vi "Aux2 IO.vi"() -> ()   [LabVIEW 2020]
uses:
  <vilib>/Platform/TimedLoop/XDataNode/timing_clust.ctl
  <vilib>/Platform/TimedLoop/XDataNode/nitl_modes.ctl
  <vilib>/Platform/TimedLoop/XDataNode/wakeup.ctl
  <vilib>/rvi/Emulation/niFpgaGetClockAttributes.vi
  <vilib>/rvi/Emulation/niFpgaSctlEmulationGetInTimedLoop.vi
  <vilib>/rvi/Emulation/niFpgaEmulationReportErrorSimple.vi
  <vilib>/rvi/eio/common/nirviEmuTemplateMethod_errors.vi
  <vilib>/rvi/Emulation/niFpgaProcessEmulError.vi
  <vilib>/rvi/Emulation/niFpgaCriticalErrorInLSC.vi
  <vilib>/eio/EIONode/EIONode.xnode
  <vilib>/platform/TimedLoop/XDataNode/XDataNode.xnode
  <vilib>/Platform/TimedLoop/XDataNode/XDNodeRunTimeDep.lvlib
  Front Panel Globals.vi
panel:
  out "Universal Data":sgl[](array[numeric])
  out "Universal Looprate":sgl
  out "TC Data":sgl[](array[numeric])
  out "TC Looprate":sgl
  out "RTD Data":sgl[](array[numeric])
  out "RTD Looprate":sgl
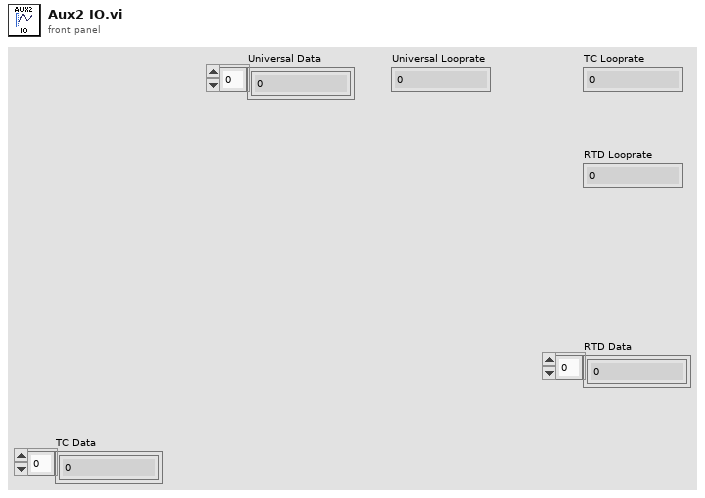
[diagram p1: front panel]
types:
  T1 = typedef "XDNodeRunTimeDep.lvlib/timing_clust.ctl" = cluster{"Expected End [f-1]":u64, "Actual End [f-1]":u64, "Finished Late? [f-1]":bool, "Expected End [i-1]":u64, "Actual End [i-1]":u64, "Finished Late? [i-1]":bool, "Expected Start [i]":u64, "Actual Start [i]":u64, "Expected Start [f]":u64, "Actual Start [f]":u64, "Source Name":string, "Structure Name":string, "Period":i64, "Deadline":i64, "Offset":i64, "Start":i64, "Priority":i32, "Timeout":i32, "Mode":T2, "Wakeup Reason":T3, "Error":errorcluster, "Source Type":string, "Secondary Source Type":string, "Global End Time":u64, "Global Start Time":u64, "Frame Duration":u64, "Iteration Duration":u64, "Assigned CPU":i32, "I/O Scan Engine Mode":u32}
  T2 = typedef "XDNodeRunTimeDep.lvlib/nitl_modes.ctl" = enum32{"No Change", "Process missed periods, maintain original phase", "Discard missed periods, maintain original phase", "Process missed periods, ignore original phase", "Discard missed periods, ignore original phase"}
  T3 = typedef "XDNodeRunTimeDep.lvlib/wakeup.ctl" = enum32{"Normal", "Aborted", "Asynchronous wakeup", "Timing source error", "Timed loop error", "Timeout"}
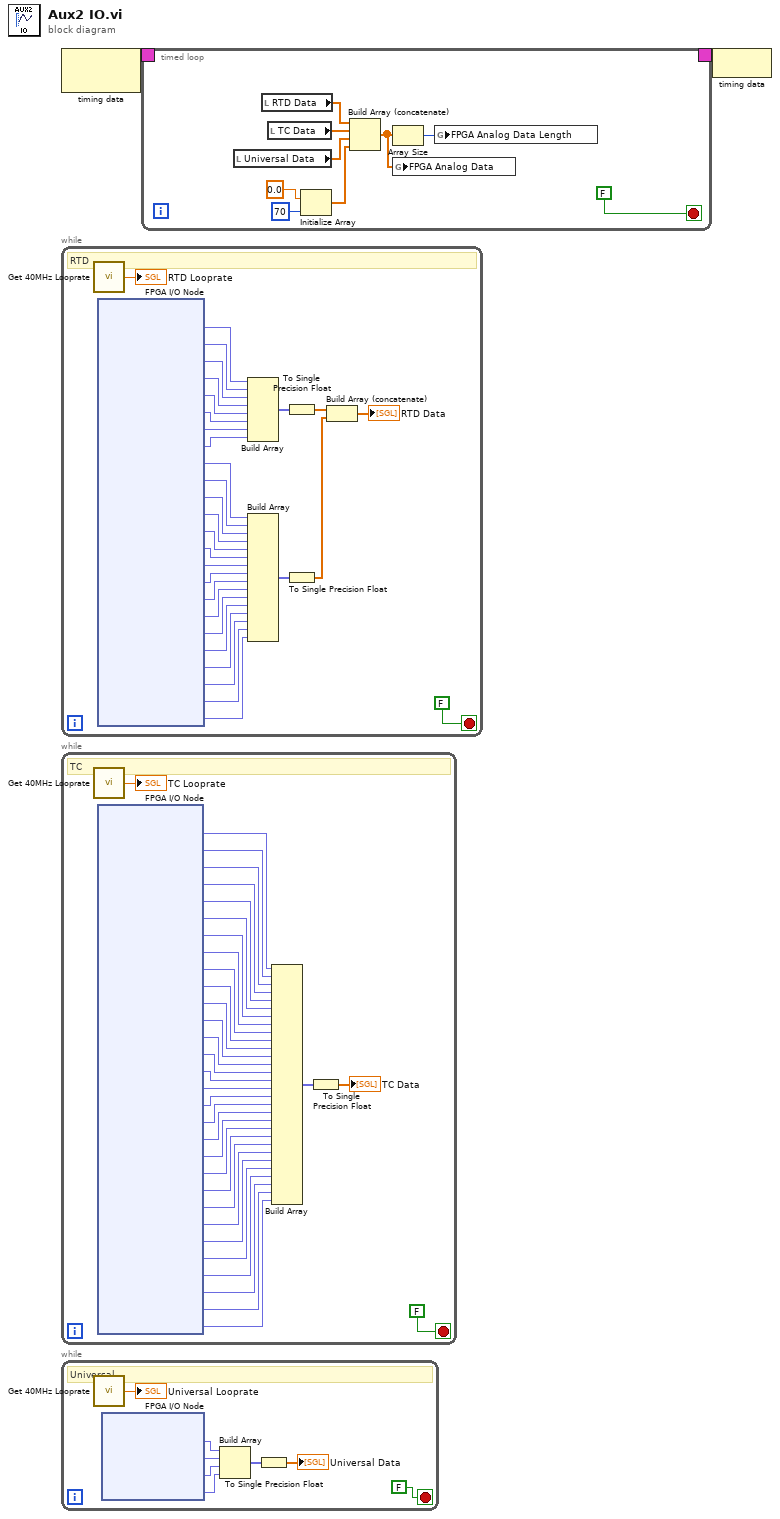
[diagram p0: block diagram]
diagram:
  n1 = node-c288() -> (w2:T1)  [unwired: 1 in]
  n2 = while {
    stop <- FALSE stop-if-true
    # "RTD"
    n3 = call "Get 40MHz Looprate.vi"() -> ("Looprate"=→"RTD Looprate":sgl)  [unwired: 5 in]
    n4 = xnode "FPGA I/O Node"() -> ("Mod1/RTD0"=w31:fxp<+/-,24,10>, "Mod1/RTD1"=w30:fxp<+/-,24,10>, "Mod1/RTD2"=w29:fxp<+/-,24,10>, "Mod1/RTD3"=w28:fxp<+/-,24,10>, "Mod1/RTD4"=w27:fxp<+/-,24,10>, "Mod1/RTD5"=w26:fxp<+/-,24,10>, "Mod1/RTD6"=w25:fxp<+/-,24,10>, "Mod1/RTD7"=w24:fxp<+/-,24,10>, "Mod2/RTD0"=w23:fxp<+/-,24,14>, "Mod2/RTD1"=w22:fxp<+/-,24,14>, "Mod2/RTD2"=w21:fxp<+/-,24,14>, "Mod2/RTD3"=w20:fxp<+/-,24,14>, "Mod2/RTD4"=w19:fxp<+/-,24,14>, "Mod2/RTD5"=w18:fxp<+/-,24,14>, "Mod2/RTD6"=w17:fxp<+/-,24,14>, "Mod2/RTD7"=w16:fxp<+/-,24,14>, "Mod3/RTD0"=w15:fxp<+/-,24,14>, "Mod3/RTD1"=w14:fxp<+/-,24,14>, "Mod3/RTD2"=w13:fxp<+/-,24,14>, "Mod3/RTD3"=w12:fxp<+/-,24,14>, "Mod3/RTD4"=w11:fxp<+/-,24,14>, "Mod3/RTD5"=w10:fxp<+/-,24,14>, "Mod3/RTD6"=w9:fxp<+/-,24,14>, "Mod3/RTD7"=w8:fxp<+/-,24,14>)  [unwired: 24 in, 24 out]
    n5 = Build Array(w31, w30, w29, w28, w27, w26, w25, w24) -> (w5:fxp<+/-,24,10>[])
    n6 = Build Array(w23, w22, w21, w20, w19, w18, w17, w16, w15, w14, w13, w12, w11, w10, w9, w8) -> (w7:fxp<+/-,24,14>[])
    n7 = To Single Precision Float(number=w5) -> (single precision float=w4:sgl[])
    n8 = To Single Precision Float(number=w7) -> (single precision float=w6:sgl[])
    n9 = Build Array (concatenate)(w4, w6) -> (→"RTD Data":sgl[])
  }
  n10 = while {
    stop <- FALSE stop-if-true
    # "TC"
    n11 = call "Get 40MHz Looprate.vi"() -> ("Looprate"=→"TC Looprate":sgl)  [unwired: 5 in]
    n12 = xnode "FPGA I/O Node"() -> ("Mod4/TC0"=w65:fxp<+/-,24,-2>, "Mod4/TC1"=w63:fxp<+/-,24,-2>, "Mod4/TC2"=w62:fxp<+/-,24,-2>, "Mod4/TC3"=w61:fxp<+/-,24,-2>, "Mod4/TC4"=w60:fxp<+/-,24,-2>, "Mod4/TC5"=w59:fxp<+/-,24,-2>, "Mod4/TC6"=w58:fxp<+/-,24,-2>, "Mod4/TC7"=w57:fxp<+/-,24,-2>, "Mod4/CJC0"=w56:fxp<+/-,24,-2>, "Mod4/CJC1"=w55:fxp<+/-,24,-2>, "Mod5/TC0"=w54:fxp<+/-,24,-2>, "Mod5/TC1"=w53:fxp<+/-,24,-2>, "Mod5/TC2"=w52:fxp<+/-,24,-2>, "Mod5/TC3"=w51:fxp<+/-,24,-2>, "Mod5/TC4"=w50:fxp<+/-,24,-2>, "Mod5/TC5"=w49:fxp<+/-,24,-2>, "Mod5/TC6"=w48:fxp<+/-,24,-2>, "Mod5/TC7"=w47:fxp<+/-,24,-2>, "Mod5/CJC0"=w46:fxp<+/-,24,-2>, "Mod5/CJC1"=w45:fxp<+/-,24,-2>, "Mod6/TC0"=w44:fxp<+/-,24,-2>, "Mod6/TC1"=w43:fxp<+/-,24,-2>, "Mod6/TC2"=w42:fxp<+/-,24,-2>, "Mod6/TC3"=w41:fxp<+/-,24,-2>, "Mod6/TC4"=w40:fxp<+/-,24,-2>, "Mod6/TC5"=w39:fxp<+/-,24,-2>, "Mod6/TC6"=w38:fxp<+/-,24,-2>, "Mod6/TC7"=w37:fxp<+/-,24,-2>, "Mod6/CJC0"=w36:fxp<+/-,24,-2>, "Mod6/CJC1"=w35:fxp<+/-,24,-2>)  [unwired: 30 in, 30 out]
    n13 = Build Array(w65, w63, w62, w61, w60, w59, w58, w57, w56, w55, w54, w53, w52, w51, w50, w49, w48, w47, w46, w45, w44, w43, w42, w41, w40, w39, w38, w37, w36, w35) -> (w64:fxp<+/-,24,-2>[])
    n14 = To Single Precision Float(number=w64) -> (single precision float=→"TC Data":sgl[])
  }
  n15 = while {
    stop <- FALSE stop-if-true
    # "Universal"
    n16 = call "Get 40MHz Looprate.vi"() -> ("Looprate"=→"Universal Looprate":sgl)  [unwired: 5 in]
    n17 = xnode "FPGA I/O Node"() -> ("Mod7/CH0"=w73:fxp<+/-,32,7>, "Mod7/CH1"=w71:fxp<+/-,32,7>, "Mod7/CH2"=w70:fxp<+/-,32,7>, "Mod7/CH3"=w69:fxp<+/-,32,7>)  [unwired: 4 in, 4 out]
    n18 = Build Array(w73, w71, w70, w69) -> (w72:fxp<+/-,32,7>[])
    n19 = To Single Precision Float(number=w72) -> (single precision float=→"Universal Data":sgl[])
  }
  n20 = timed-loop {
    timing: w2 -> [_]
    timing-out: [_] -> w1
    stop <- FALSE stop-if-true
    n21 = local read "Universal Data"() -> (w81:sgl[])
    n22 = local read "RTD Data"() -> (w83:sgl[])
    n23 = local read "TC Data"() -> (w82:sgl[])
    n24 = Initialize Array(sgl 0.0 ("element"), 70 ("dimension size")) -> (w77:sgl[])
    n25 = Build Array (concatenate)(w83, w82, w81, w77) -> (w80:sgl[])
    n26 = Array Size(array=w80) -> (size(s)=w76:i32)
    n27 = global write "Front Panel Globals.vi" "FPGA Analog Data"(w80) -> ()
    n28 = global write "Front Panel Globals.vi" "FPGA Analog Data Length"(w76) -> ()
  }
  n29 = node-c288(w1) -> ()
